vi "Read LNA Status.vi"(11 "Test LNA in":refnum<class "TestLNA.lvclass">) -> (2 "LNA Status":T1, 3 "Test LNA out":refnum<class "TestLNA.lvclass">)   [LabVIEW 2014, in "TestLNA.lvlib" / "TestLNA.lvclass"]
uses:
  TestLNA.lvclass
  TestLNA.lvclass/TestLNA.ctl
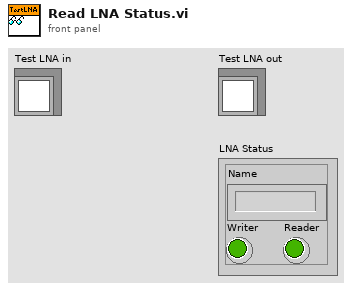
[diagram p1: front panel]
types:
  T1 = cluster{"Name":string, "Writer":bool, "Reader":bool}
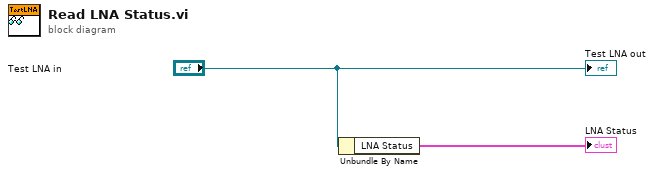
[diagram p0: block diagram]
diagram:
  n1 = Unbundle By Name("Test LNA in") -> ("LNA Status"=→"LNA Status":T1)
  "Test LNA out" <- "Test LNA in"
